vi "Create Color Table.vi"() -> (2 "Color Table":u32[](array[numeric]), 3 "Array":T1(array[cluster]))   [LabVIEW 2022 SP3]
doc: "Demonstrates how to interactively and programmatically modify the color table for an intensity graph or intensity chart."
panel:
  in  "Doppler":u32[](array[colorbox])=[8454143, 1970943, 0, 16711680, 16776960]
  out "Intensity Graph":dbl[][](graph)
  # "Overview: Demonstrates how to interactively and programmatically modify the Color Table of an Intensity Graph or Intensity Chart.\nInstructions:\n1. Run the VI.\n2. Right-click one of the numbers on the Z Scale (the color ramp on the right side of the graph) and choose Marker Color to interactively change the color associated with that scale marker.  Observe the color change, and that the rest of the color ramp interpolates according to the new color.\n3. Click the Update Marker Colors button to programmatically apply new colors to the three markers on the Z Scale.\n4. Click Stop to stop the VI."
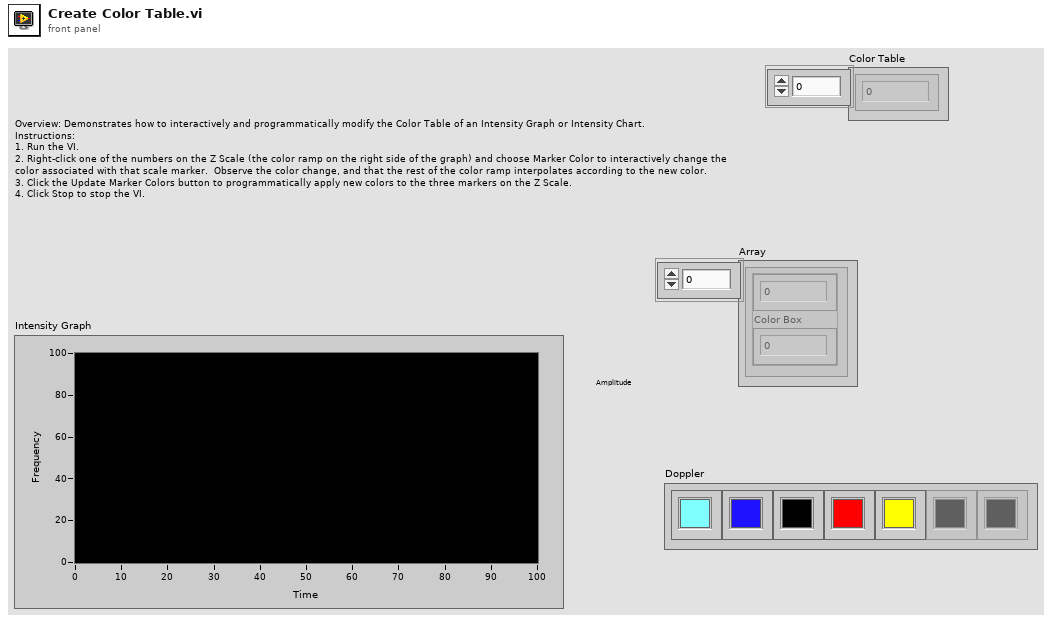
[diagram p1: front panel]
types:
  T1 = cluster{"Numeric Control":dbl, "Color Box":u32}[]
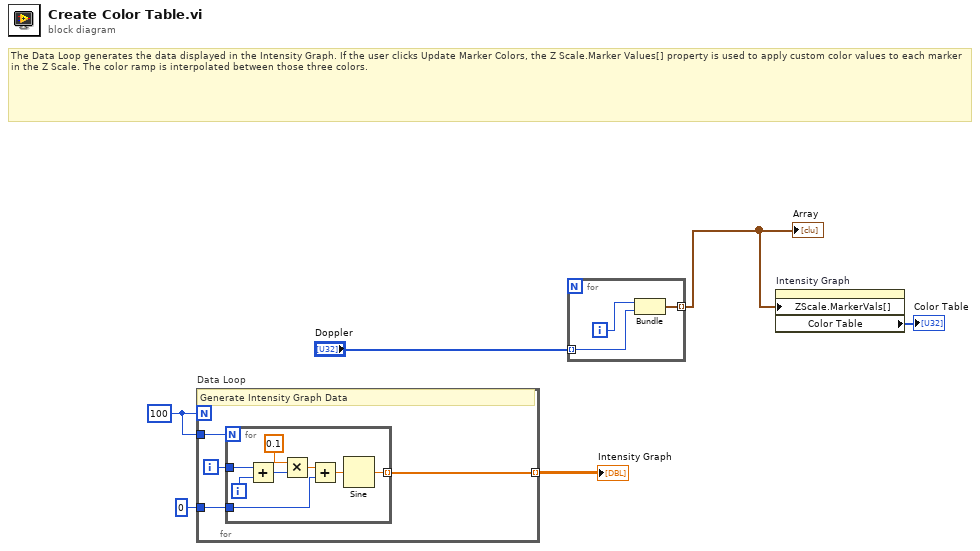
[diagram p0: block diagram]
diagram:
  w6 = 100
  # "The Data Loop generates the data displayed in the Intensity Graph. If the user clicks Update Marker Colors, the Z Scale.Marker Values[] property is used to apply custom color values to each marker in the Z Scale. The color ramp is interpolated between those three colors."
  n1 = for "Data Loop" {
    N: w6 -> [_]
    tunnel: [w10] -> w2 mode=indexing
    tunnel: w6 -> [w9]
    tunnel: 0 -> [w7]
    i -> [w8]
    # "Generate Intensity Graph Data"
    n2 = for {
      N: w9 -> [_]
      tunnel: [w18] -> w10 mode=indexing
      tunnel: w8 -> [w15]
      tunnel: w7 -> [w11]
      i -> [w16]
      n3 = Add(x=w15, y=w16) -> (x+y=w17:i32)
      n4 = Multiply(x=0.1, y=w17) -> (x*y=w14:dbl)
      n5 = Add(x=w14, y=w11) -> (x+y=w12:dbl)
      n6 = Sine(x=w12) -> (sin(x)=w18:dbl)
    }
  }
  "Intensity Graph" <- w2
  n7 = for {
    tunnel: "Doppler" -> [w21] mode=indexing
    tunnel: [w20] -> w3 mode=indexing
    i -> [w19]
    n8 = Bundle(w19, "Color Box"=w21) -> (w20:cluster{i32, "Color Box":u32})  [unwired: 1 in]
  }
  "Array" <- w3
  n9 = property on="Intensity Graph" class="IntensityGraph (strict)"("ZScale.MarkerVals[]"=w3) -> ("Color Table"=→"Color Table":u32[])  [unwired: 2 in, 2 out]
